vi "DSF.Engine.Memory.Cache.Transfer Group.Get Largest Count.All Types.vi"(8 "error in (no error)":errorcluster, 10 "Data Type Counts in":T1 {"U64" format="%d elements"; "U32" format="%d elements"; "U16" format="%d elements"; "U8" format="%d elements"; "I64" format="%d elements"; "I32" format="%d elements"; "I16" format="%d elements"; "I8" format="%d elements"; "DBL" format="%d elements"; "SGL" format="%d elements"; "Bool" format="%d elements"}, 11 "Transfer Group Cache in":refnum<class "DSF.Engine.Memory.Cache.Transfer Group.lvclass">) -> (0 "error out":errorcluster, 2 "Data Type Counts out":T1 {"U64" format="%d elements"; "U32" format="%d elements"; "U16" format="%d elements"; "U8" format="%d elements"; "I64" format="%d elements"; "I32" format="%d elements"; "I16" format="%d elements"; "I8" format="%d elements"; "DBL" format="%d elements"; "SGL" format="%d elements"; "Bool" format="%d elements"}, 3 "Transfer Group Cache out":refnum<class "DSF.Engine.Memory.Cache.Transfer Group.lvclass">)   [LabVIEW 2016, in "DSF.Engine.lvlib" / "DSF.Engine.Memory.Cache.Transfer Group.lvclass"]
uses:
  DSF.Engine.Memory.Cache.Transfer Group.lvclass
  Shared/Typedefs/DSF.Shared.Typedefs.Data Type Counts.ctl
  DSF.Engine.Memory.Cache.Transfer Group.lvclass/DSF.Engine.Memory.Cache.Transfer Group.ctl
  DSF.Engine.Memory.Cache.Transfer.lvclass/DSF.Engine.Memory.Cache.Transfer.ctl
  Shared/Classes/Transfer/DSF.Shared.Configuration.Transfer.lvclass/DSF.Shared.Configuration.Transfer.ctl
  DSF.Engine.Memory.Cache.Transfer.Get Configuration.vi
  Shared/Classes/Transfer/DSF.Shared.Configuration.Transfer.Get Block Descriptors.vi
  DSF.Engine.Memory.Cache.Transfer.lvclass
  DSF.Shared.lvlib
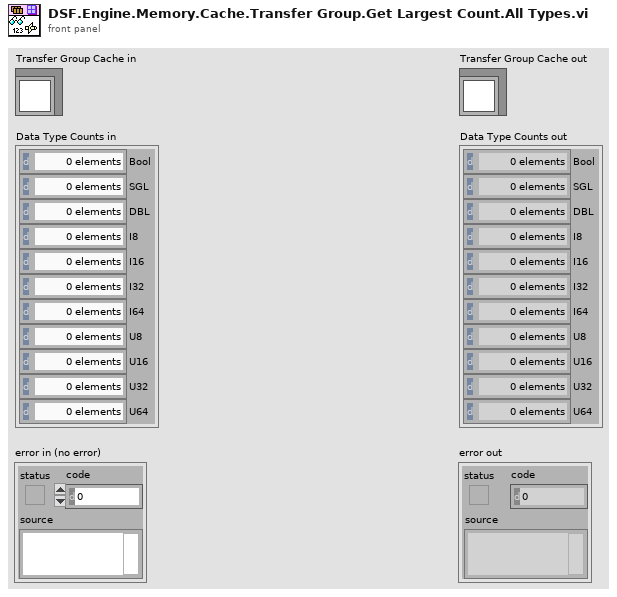
[diagram p1: front panel]
types:
  T1 = typedef "DSF.Shared.lvlib/DSF.Shared.Typedefs.Data Type Counts.ctl" = cluster{"Bool":u64, "SGL":u64, "DBL":u64, "I8":u64, "I16":u64, "I32":u64, "I64":u64, "U8":u64, "U16":u64, "U32":u64, "U64":u64}
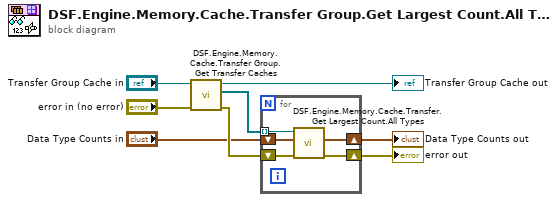
[diagram p0: block diagram]
diagram:
  n1 = call "DSF.Engine.Memory.Cache.Transfer Group.Get Transfer Caches.vi"("error in (no error)"="error in (no error)", "Transfer Group Cache in"="Transfer Group Cache in") -> ("error out"=w4:errorcluster, "Transfer Caches"=w6:refnum<class "DSF.Engine.Memory.Cache.Transfer.lvclass">[], "Transfer Group Cache out"=→"Transfer Group Cache out":refnum<class "DSF.Engine.Memory.Cache.Transfer Group.lvclass">)  [unwired: 7 in]
  n2 = for {
    tunnel: w6 -> [w13] mode=indexing
    shift-right: [w12] -> w5
    shift-left: w4 -> [w11]
    shift-right: [w10] -> w1
    shift-left: "Data Type Counts in" -> [w9]
    n3 = call "DSF.Engine.Memory.Cache.Transfer.Get Largest Count.All Types.vi"("error in (no error)"=w11, "Data Type Counts in"=w9, "Transfer Cache in"=w13) -> ("error out"=w12:errorcluster, "Data Type Counts out"=w10:T1)  [unwired: 6 in, 1 out]
  }
  "error out" <- w5
  "Data Type Counts out" <- w1
